vi "FileUpToDate.vi"(1 "FileUpToDate in":bool caption="Parameter Changed", 4 "DIMControSet out":refnum<vi>[](array[refnum]), 5 "CtlRef":refnum<vi>) -> (15 "FileUpToDate out":bool caption="Parameter Changed")   [LabVIEW 2014, in "Panels.lvlib"]
uses:
  Panels.lvlib
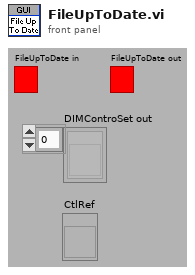
[diagram p1: front panel]
types:
  T1 = cluster{"data":dbl[], "no link":bool, "quality":i32, "timeStamp":dbl}
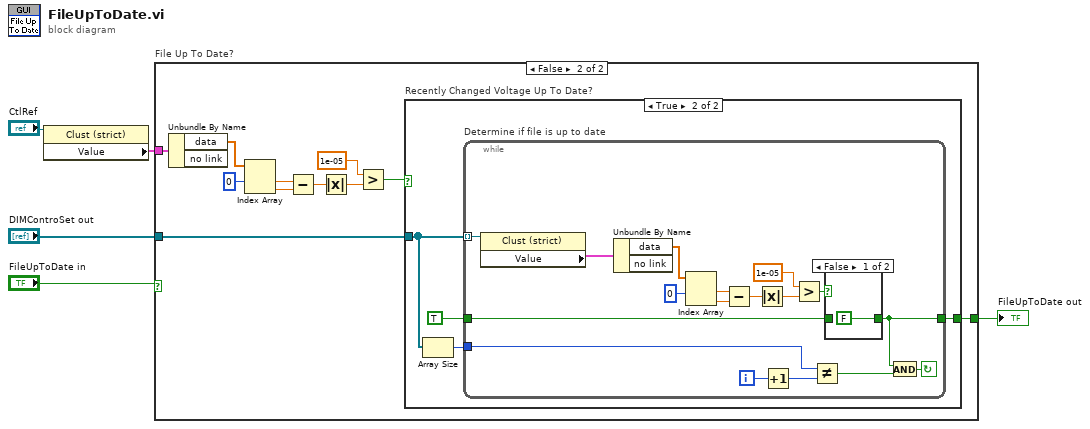
[diagram p0: block diagram]
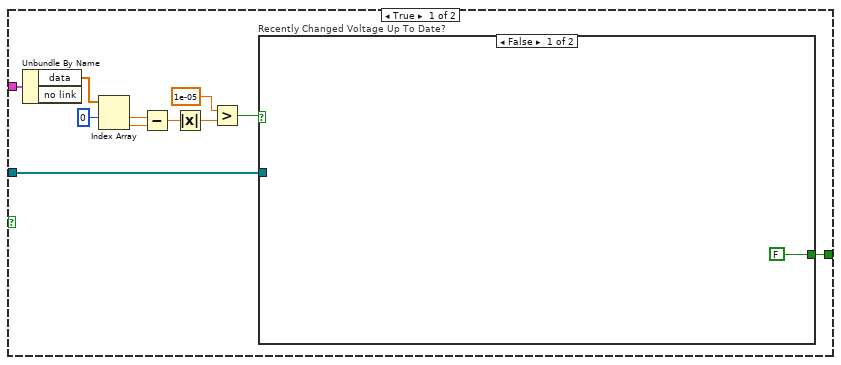
[diagram p2: hidden frame]
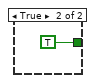
[diagram p3: hidden frame]
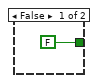
[diagram p4: hidden frame]
diagram:
  n1 = property class="Clust (strict)"(reference="CtlRef") -> ("Value"=w1:T1)  [unwired: 1 in, 2 out]
  n2 = case "File Up To Date?" shown="False" "FileUpToDate in" {
    tunnel: "DIMControSet out" -> [w16 w29]
    tunnel: [w15 w28] -> w4
    tunnel: w1 -> [w12 w25]
    frame True {
      n3 = Unbundle By Name(w12) -> ("data"=w13:dbl[])  [unwired: 1 out]
      n4 = Index Array(array=w13, index #1=0 ("index")) -> (element #1=w11:dbl, element #2=w10:dbl)  [unwired: 1 in]
      n5 = Subtract(x=w11, y=w10) -> (x-y=w9:dbl)
      n6 = Absolute Value(x=w9) -> (abs(x)=w8:dbl)
      n7 = Greater?(x=1e-05, y=w8) -> (0:w6:bool)
      n8 = case "Recently Changed Voltage Up To Date?" shown="False" w6 {
        tunnel: w16 -> [_ _]
        tunnel: [FALSE ("FileUpToDate") TRUE ("FileUpToDate")] -> w15
        frame False {
        }
        frame True {
        }
      }
    }
    frame False {
      n9 = Unbundle By Name(w25) -> ("data"=w26:dbl[])  [unwired: 1 out]
      n10 = Index Array(array=w26, index #1=0 ("index")) -> (element #1=w24:dbl, element #2=w23:dbl)  [unwired: 1 in]
      n11 = Subtract(x=w24, y=w23) -> (x-y=w22:dbl)
      n12 = Absolute Value(x=w22) -> (abs(x)=w21:dbl)
      n13 = Greater?(x=1e-05, y=w21) -> (0:w19:bool)
      n14 = case "Recently Changed Voltage Up To Date?" shown="True" w19 {
        tunnel: w29 -> [_ w32]
        tunnel: [FALSE ("FileUpToDate") w34] -> w28
        frame False {
        }
        frame True {
          n15 = Array Size(array=w32) -> (size(s)=w31:i32)
          n16 = while "Determine if file is up to date" {
            tunnel: w32 -> [w51] mode=indexing
            tunnel: [w39] -> w34
            tunnel: TRUE ("FileUpToDate") -> [w44]
            tunnel: w31 -> [w36]
            i -> [w38]
            stop <- w40 continue-if-true
            n17 = property class="Clust (strict)"(reference=w51) -> ("Value"=w48:T1)  [unwired: 1 in, 2 out]
            n18 = Unbundle By Name(w48) -> ("data"=w49:dbl[])  [unwired: 1 out]
            n19 = Index Array(array=w49, index #1=0 ("index")) -> (element #1=w43:dbl, element #2=w42:dbl)  [unwired: 1 in]
            n20 = Subtract(x=w43, y=w42) -> (x-y=w47:dbl)
            n21 = Absolute Value(x=w47) -> (abs(x)=w46:dbl)
            n22 = Increment(x=w38) -> (x+1=w37:i32)
            n23 = Greater?(x=1e-05, y=w46) -> (0:w41:bool)
            n24 = Not Equal?(x=w36, y=w37) -> (x != y?=w35:bool)
            n25 = case shown="False" w41 {
              tunnel: [FALSE ("FileUpToDate") w53] -> w39
              tunnel: w44 -> [_ w53]
              frame False {
              }
              frame True {
              }
            }
            n26 = And(x=w39, y=w35) -> (x .and. y?=w40:bool)
          }
        }
      }
    }
  }
  "FileUpToDate out" <- w4
